vi "Basic Read Busy Flag and Address.vi"(6 "chip select  (1st chip)":enum16{"1st chip", "2nd chip"}(ring), 8 "error in (no error)":errorcluster, 11 "cluster of private data in":T1={"FPGA VI Reference"=refnum, "device index"=0, "screen size"=enum."8x1", "font size"=enum."5x8", "auto wrap"=FALSE, "alignment"=enum."None", "number of line"=enum."2 lines", "shift 0"=0, "entry mode 0"=enum."increment & no shift", "shift 1"=0, "entry mode 1"=enum."increment & no shift"}) -> (0 "error out":errorcluster, 1 "address":u8=97 format="%.0x", 2 "busy flag":bool, 3 "cluster of private data out":T1={"FPGA VI Reference"=refnum, "device index"=0, "screen size"=enum."8x1", "font size"=enum."5x8", "auto wrap"=FALSE, "alignment"=enum."None", "number of line"=enum."2 lines", "shift 0"=0, "entry mode 0"=enum."increment & no shift", "shift 1"=0, "entry mode 1"=enum."increment & no shift"})   [LabVIEW 2017, in "HD44780.lvclass"]
uses:
  HD44780.lvclass
  Common/HD44780 Common.lvlib
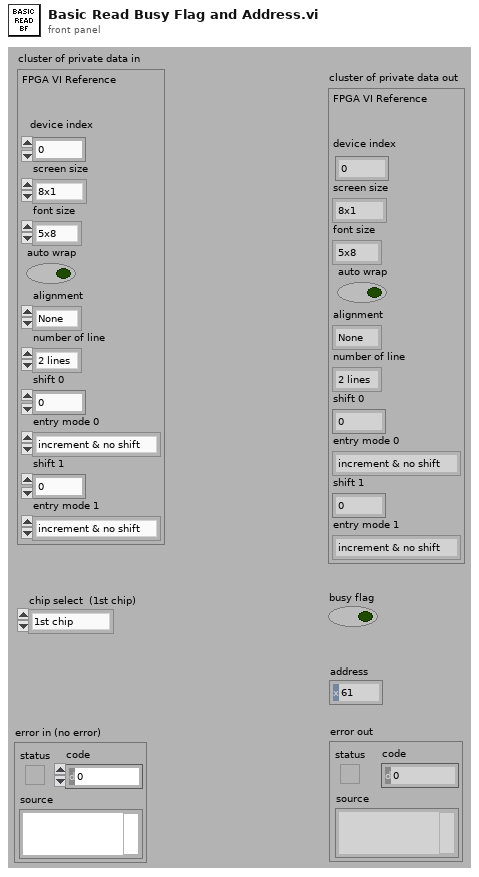
[diagram p1: front panel]
types:
  T1 = cluster{"FPGA VI Reference":refnum<k20>, "device index":i8, "screen size":enum8{"8x1", "8x2", "12x4", "16x1", "16x2", "16x4", "20x1", "20x2", "20x4", "24x1", "24x2", "40x2", "40x4"}, "font size":enum8{"5x8", "5x10"}, "auto wrap":bool, "alignment":enum16{"None", "Left", "Center", "Right"}, "number of line":enum8{"1 line", "2 lines"}, "shift 0":i8, "entry mode 0":enum8{"increment & no shift", "increment & shift", "decrement & no shift", "decrement & shift"}, "shift 1":i8, "entry mode 1":enum8{"increment & no shift", "increment & shift", "decrement & no shift", "decrement & shift"}}
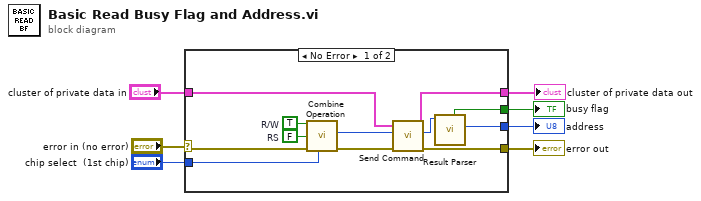
[diagram p0: block diagram]
diagram:
  n1 = case shown="No Error" "error in (no error)" {
    selector: "error in (no error)" -> [w8 w21]
    tunnel: [w14 w21] -> w5
    tunnel: [w18 _] -> w7
    tunnel: [w17 _] -> w6
    tunnel: "chip select  (1st chip)" -> [w10 _]
    tunnel: "cluster of private data in" -> [w9 w20]
    tunnel: [w11 w20] -> w1
    frame No Error {
      w12 = FALSE  # RS
      w19 = TRUE  # R/W
      n2 = call "Combine Operation.vi"("chip select  (1st chip)"=w10, "error in (no error)"=w8, "RS"=w12, "R/W"=w19) -> ("error out"=w16:errorcluster, "output"=w13:u32)  [unwired: 6 in]
      n3 = call "Send Command.vi"("error in (no error)"=w16, "operation"=w13, "cluster of private data in"=w9) -> ("error out"=w14:errorcluster, "result"=w15:u32, "cluster of private data out"=w11:T1)  [unwired: 6 in]
      n4 = call "Result Parser.vi"("operation"=w15) -> ("address"=w17:u8, "busy flag"=w18:bool)  [unwired: 8 in, 1 out]
    }
    frame Error {
    }
  }
  "error out" <- w5
  "busy flag" <- w7
  "address" <- w6
  "cluster of private data out" <- w1
